vi "Trigger Multiplexer.vi"(7 "Trigger Type":T1(ring)=enum."Software Trigger", 8 "Analog Trigger":bool, 9 "Digital Trigger":bool, 10 "Software Trigger":bool, 11 "Immediate Trigger":bool) -> (2 "Trigger Out":bool)   [LabVIEW 2012]
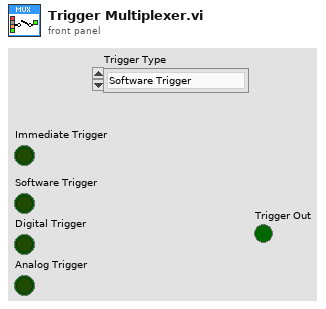
[diagram p1: front panel]
types:
  T1 = enum8{"Immediate Trigger", "Software Trigger", "External Digital Trigger", "Analog Trigger"}
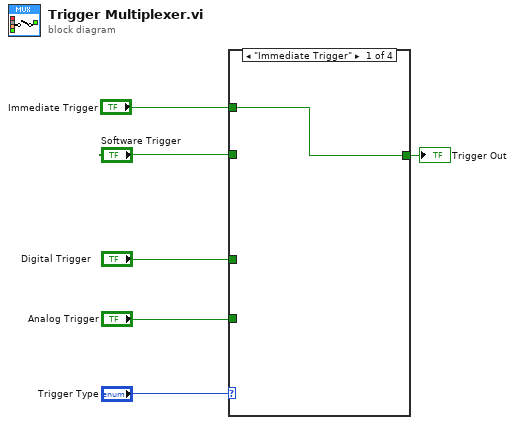
[diagram p0: block diagram]
diagram:
  n1 = case shown="\"Immediate Trigger\"" "Trigger Type" {
    tunnel: [w7 w8 w9 w10] -> w2
    tunnel: "Digital Trigger" -> [_ _ w9 _]
    tunnel: "Software Trigger" -> [_ w8 _ _]
    tunnel: "Analog Trigger" -> [_ _ _ w10]
    tunnel: "Immediate Trigger" -> [w7 _ _ _]
    frame "Immediate Trigger" {
    }
    frame "Software Trigger" {
    }
    frame "External Digital Trigger", Default {
    }
    frame "Analog Trigger" {
    }
  }
  "Trigger Out" <- w2
